vi "Validate.vi"(8 "error in":errorcluster, 11 "Copy of PCAN in":refnum<class "PCAN.lvclass">) -> (0 "error out":errorcluster, 2 "Valid?":bool, 3 "Copy of PCAN out":refnum<class "PCAN.lvclass">)   [LabVIEW 2024, in "PCAN.lvlib" / "PCAN.lvclass"]
uses:
  PCAN.lvclass
  PCAN.lvclass/PCAN.ctl
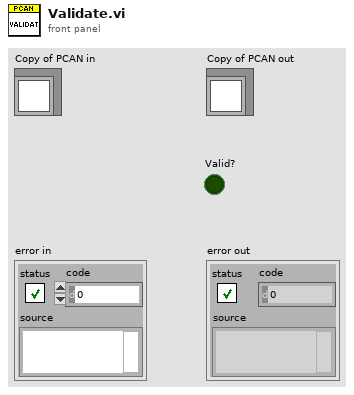
[diagram p1: front panel]
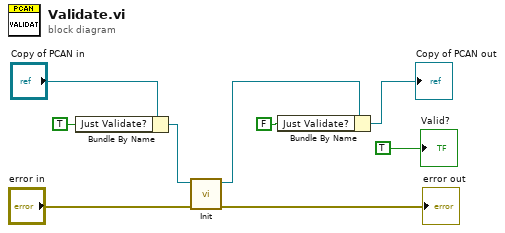
[diagram p0: block diagram]
diagram:
  n1 = Bundle By Name(cluster="Copy of PCAN in", "Just Validate?"=TRUE) -> (w5:refnum<class "PCAN.lvclass">)
  n2 = call-dynamic "Init.vi"("error in"="error in", "PCAN in"=w5) -> ("error out"=→"error out":errorcluster, "PCAN out"=w4:refnum<class "PCAN.lvclass">)  [unwired: 8 in]
  n3 = Bundle By Name(cluster=w4, "Just Validate?"=FALSE) -> (→"Copy of PCAN out":refnum<class "PCAN.lvclass">)
  "Valid?" <- TRUE ("Valid?")
